vi "lm Color Level.vi"(8 "error in (no error)":errorcluster, 10 "str_Level":string, 11 "str_Color":string) -> (0 "error out":errorcluster, 2 "str_Level out":string, 3 "str_Color out":string)   [LabVIEW 2018, in "LumencorDLL32.lvlib"]
doc: "This Function Sets the Color Level. Valid Colors are LE dependent. Color names should be in UPPER case (RED, GREEN etc.) Level is a an integer perctent value between 0 and 100.\n\n\nextern \"C\" LUMENCORDLL2B_API void lmColorLevel(char *str_Color, char *str_Level);"
uses:
  LumencorDLL32.lvlib
  LumencorDLL32.dll
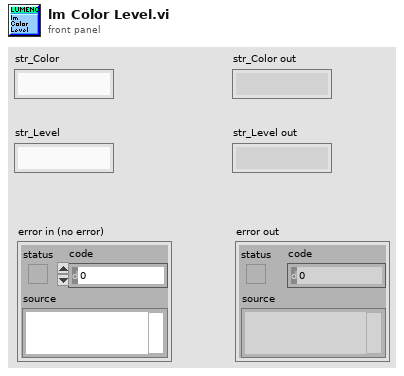
[diagram p1: front panel]
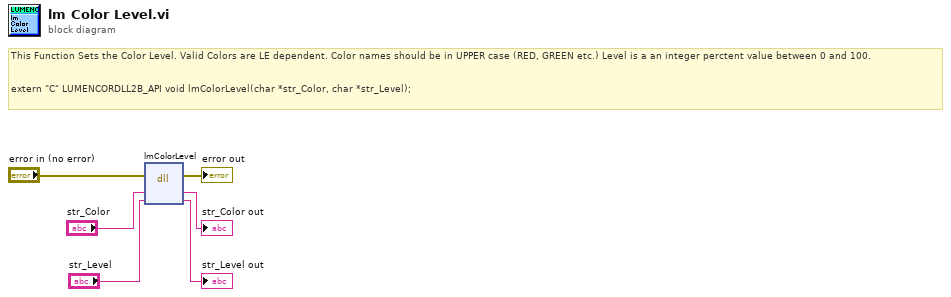
[diagram p0: block diagram]
diagram:
  # "This Function Sets the Color Level. Valid Colors are LE dependent. Color names should be in UPPER case (RED, GREEN etc.) Level is a an integer perctent value between 0 and 100.\n\n\nextern \"C\" LUMENCORDLL2B_API void lmColorLevel(char *str_Color, char *str_Level);"
  n1 = dll-call lib="C:/Users/e14user/Documents/LabVIEW software/GitRepo/lib/SOLA/LabVIEW 2015 Library (32bit)/LumencorDLL32/LumencorDLL32.*" fn="lmColorLevel"(error in="error in (no error)", "str_Color"="str_Color", "str_Level"="str_Level") -> (error out=→"error out":errorcluster, "str_Color"=→"str_Color out":string, "str_Level"=→"str_Level out":string)  [unwired: 3 in, 1 out]
